vi "Multichannel Recording0.6.vi"() -> ()   [LabVIEW 2014]
uses:
  Multichannel Record/Enum State Typedef.ctl
  <vilib>/_DAQmxBase/Internals/DAQmxBase Create Channel (AI-Voltage-Basic).vi
  <vilib>/_DAQmxBase/Internals/DAQmxBase Timing (Sample Clock).vi
  <vilib>/_DAQmxBase/Internals/DAQmxBase Read (Analog 2D DBL NChan NSamp).vi
  Consumer Data_ Consumer Event Com.ctl
  Multichannel Record/Data Producer States.ctl
panel:
  in  "Display Size":T1(ring)
  out "Total Iterations Needed":dbl
  out "Read Data":i32
  out "Data Producer State":T2=enum."Default"
  out "Data Consumer State":T3=enum."Default"
  in  "Open Button":bool
  in  "Tab Control":T4(tab)
  in  "Amplifier Channel 0":T5 {"Amplifier Model" items=["Select a Model", "AM 1700", "BMA 200"]}
  out "Channel 0 Chart":waveform(dbl)(graph)
  in  "User Data Channel 0":T6
  in  "Use Channel 0":bool caption="In Use?"
  out "Channel 1 Chart":waveform(dbl)(graph)
  in  "User Data Channel 1":T6
  in  "Amplifier Channel 1":T5 {"Amplifier Model" items=["Select a Model", "AM 1700", "BMA 200"]}
  in  "Use Channel 1":bool caption="In Use?"
  out "Channel 2 Chart":waveform(dbl)(graph)
  in  "User Data Channel 2":T6
  in  "Amplifier Channel 2":T5 {"Amplifier Model" items=["Select a Model", "AM 1700", "BMA 200"]}
  in  "Use Channel 2":bool caption="In Use?"
  out "Channel 3 Chart":waveform(dbl)(graph)
  in  "User Data Channel 3":T6
  in  "Amplifier Channel 3":T5 {"Amplifier Model" items=["Select a Model", "AM 1700", "BMA 200"]}
  in  "Use Channel 3":bool caption="In Use?"
  out "Overview Chart":waveform(dbl)[](graph)
  in  "Stop Preview":bool
  in  "OK Button":bool
  out "Event State":T7
  in  "Clear Display":bool
  in  "Preview Button":bool
  out "Iterations Recorded":i32
  in  "Recording Time (seconds)":dbl
  in  "Sample Rate":i32=1000
  in  "Stop Button":bool
  out "Start Time hr/min":string
  out "Date mm/dd/yy":string
  in  "Exit Button":bool
  in  "Record Button":bool
  # "MSU EFISH Lab Multi-Channel Electronic Pulse Recorder"
  # "Must enter numbers into here before you start"
  # "Blue for On\nOrange for Off"
  # "DC"
  # "AC"
  # "Blue for AC and Orange for DC"
  # "Blue for On\nOrange for Off"
  # "DC"
  # "AC"
  # "Blue for AC and Orange for DC"
  # "Blue for On\nOrange for Off"
  # "DC"
  # "AC"
  # "Blue for AC and Orange for DC"
  # "Blue for On\nOrange for Off"
  # "DC"
  # "AC"
  # "Blue for AC and Orange for DC"
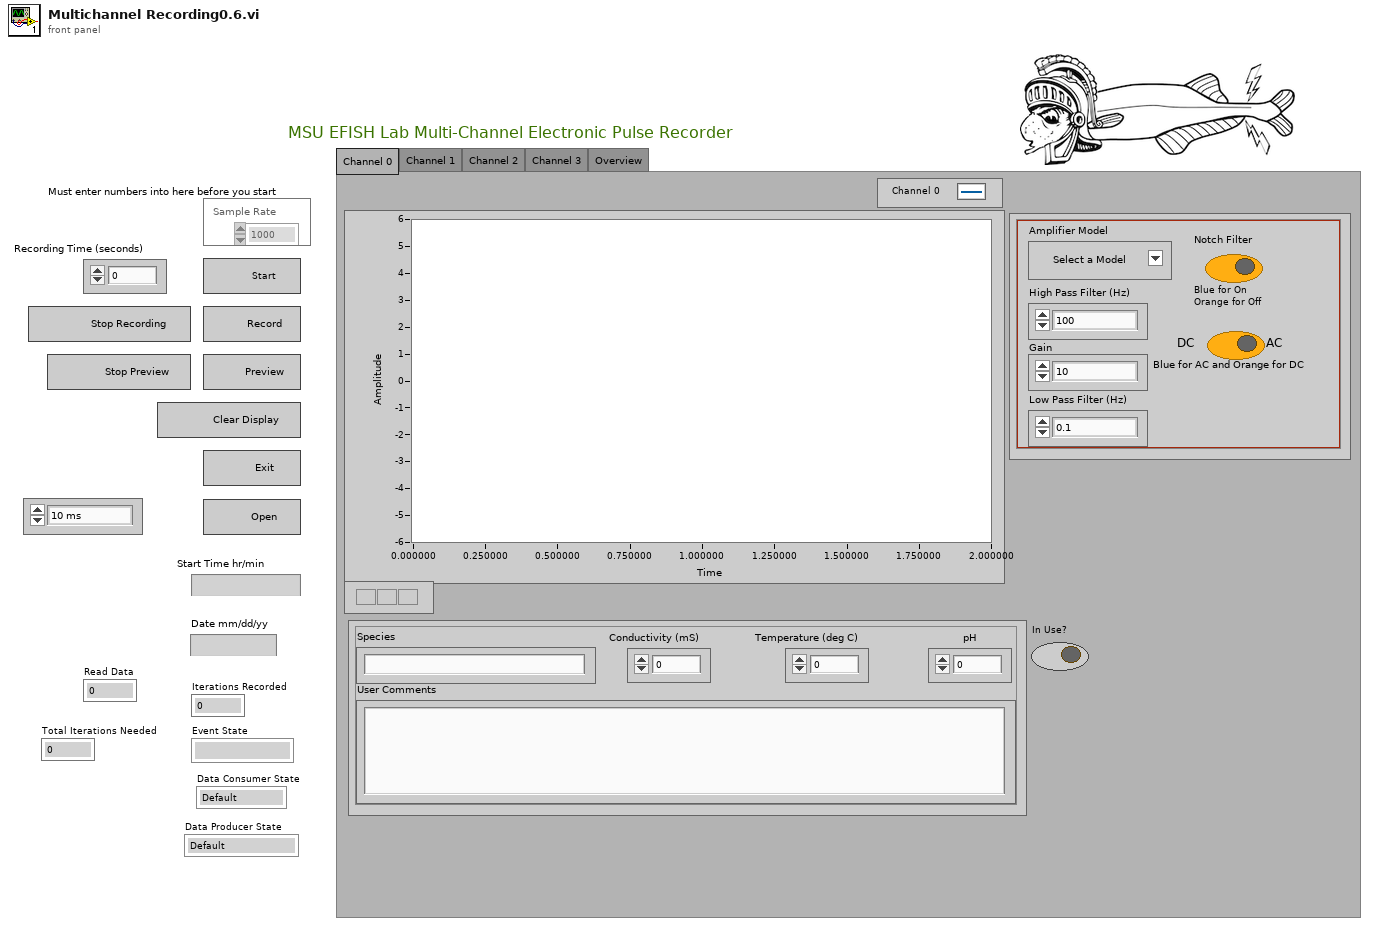
[diagram p1: front panel]
types:
  T1 = enum16{"10 ms", "100 ms", "1 Second", "10 sec", "30 sec"}
  T2 = typedef "Data Producer States.ctl" = enum16{"Read Data", "Set Sample Clock", "Default", "Exit", "Preview"}
  T3 = typedef "Consumer Data_ Consumer Event Com.ctl" = enum16{"Recording", "Create File", "Clear Memory", "Default", "End File", "Exit", "Set Sample Clock", "Preview"}
  T4 = enum32{"Channel 0", "Channel 1", "Channel 2", "Channel 3", "Overview"}
  T5 = cluster{"Low Pass Filter (Hz)":enum16{"0.1", "1", "3", "10", "30", "100", "300"}, "Gain ":enum16{"10", "20", "50", "100", "200", "500", "1000", "2k", "5k", "10k", "20k", "50k"}, "High Pass Filter (Hz)":enum16{"100", "500", "1000", "3000", "5000", "10,000", "20,000", "30,000", "50,000"}, "Notch Filter":bool, "Amplifier Model":u16, "AC/DC Switch":bool}
  T6 = cluster{"pH":dbl, "Conductivity (mS)":dbl, "Temperature (deg C)":dbl, "User Comments":string, "Species":string}
  T7 = typedef "Enum State Typedef.ctl" = enum16{"", "Open FIle", "Beginning State", "Set the Sample Clock", "Prepreview Handling", "Clear Display", "Preview Data", "Stop", "Exit", "Record", "Create File"}
  T8 = enum8{"Enabled", "Disabled", "Disabled and Grayed Out"}
  T9 = enum16{"Recording", "Create File", "Clear Memory", "Default"}
  T10 = cluster{"Refnum out":refnum<k34>, "Refnum out":refnum<k34>, "Refnum out":refnum<k34>, "Refnum out":refnum<k34>}
  T11 = cluster{"Use Channel 0":bool, "Use Channel 1":bool, "Use Channel 2":bool, "Use Channel 3":bool}
  T12 = cluster{"tdms file out":refnum<k34>, "tdms file out":refnum<k34>, "tdms file out":refnum<k34>, "tdms file out":refnum<k34>}
  T13 = cluster{"Waveform":waveform(dbl), "Waveform":waveform(dbl), "Waveform":waveform(dbl), "Waveform":waveform(dbl), waveform(dbl)[]}
  T14 = enum16{"Read Data", "Set Sample Clock", "Default", "Exit"}
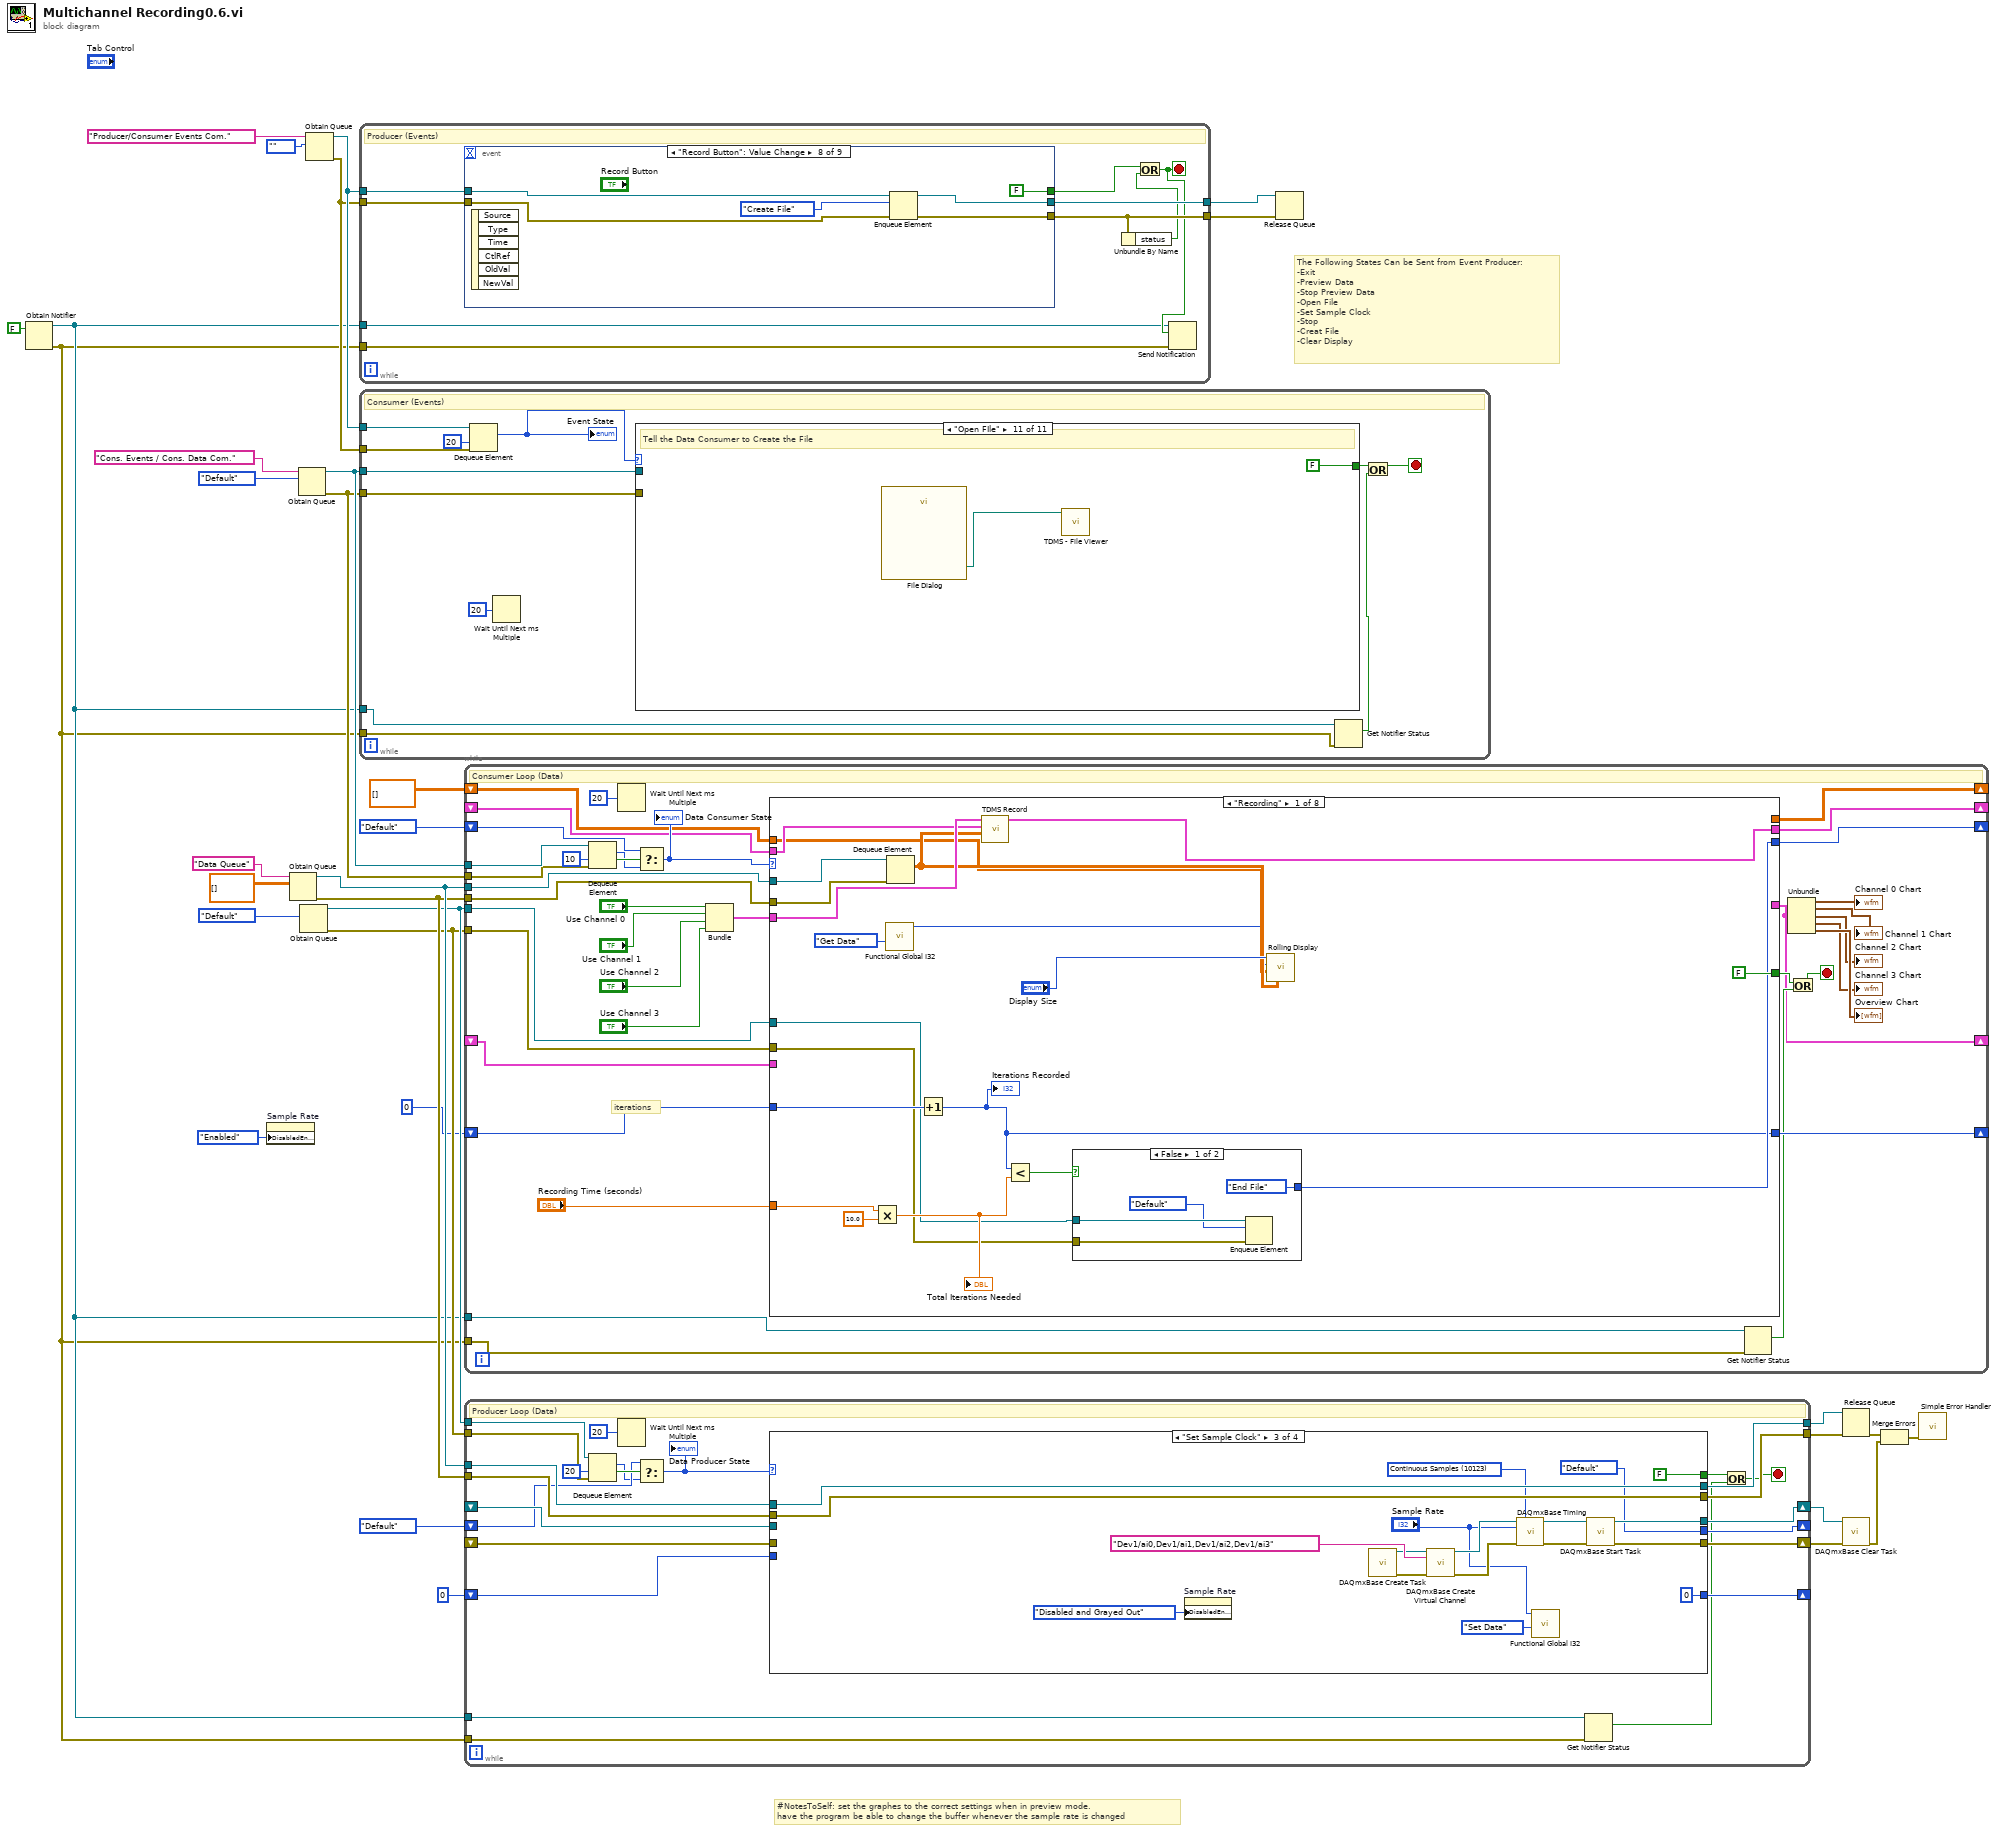
[diagram p0: block diagram]
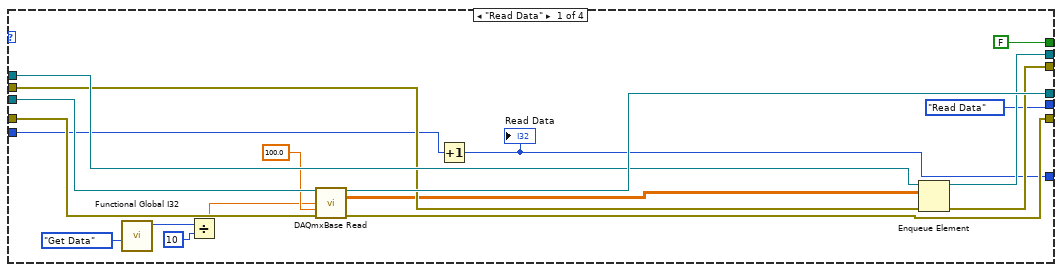
[diagram p2: hidden frame]
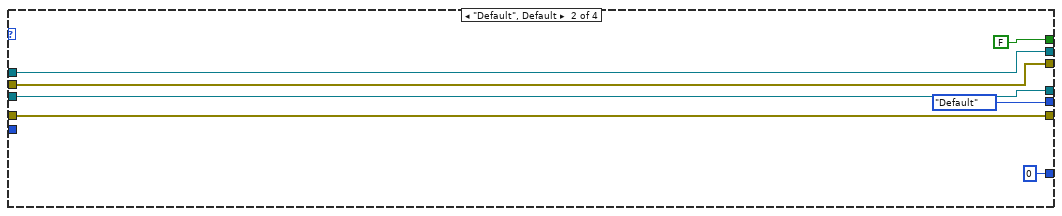
[diagram p3: hidden frame]
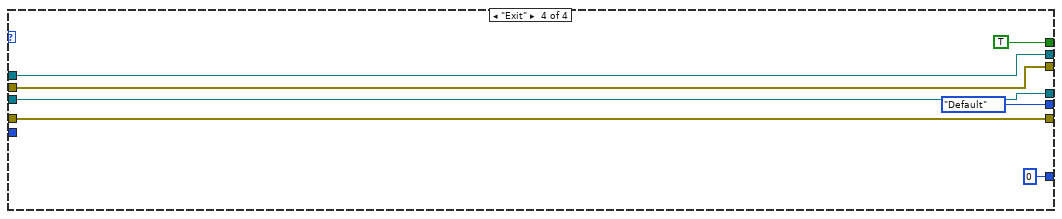
[diagram p4: hidden frame]
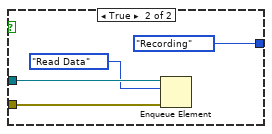
[diagram p5: hidden frame]
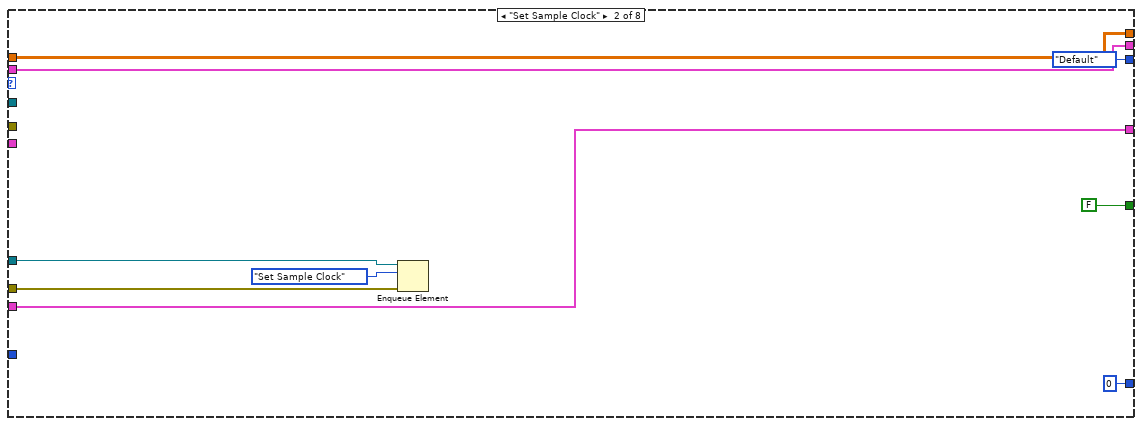
[diagram p6: hidden frame]
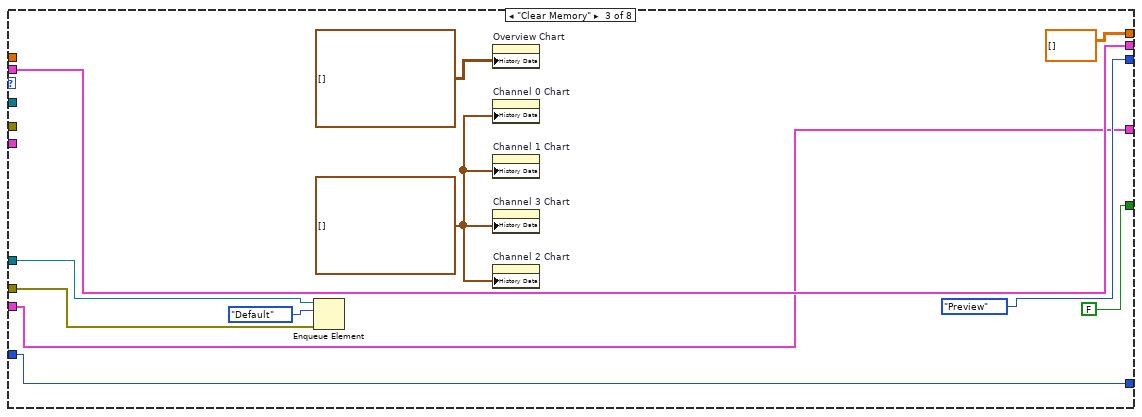
[diagram p7: hidden frame]
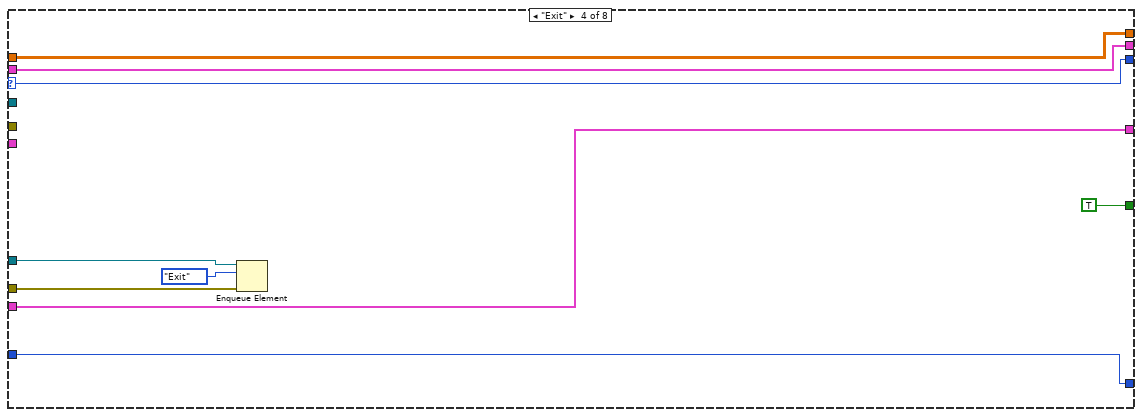
[diagram p8: hidden frame]
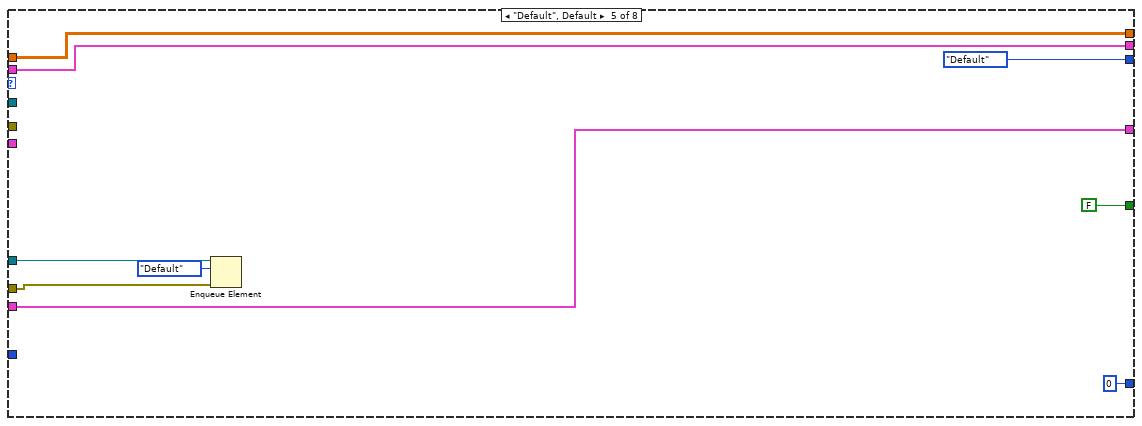
[diagram p9: hidden frame]
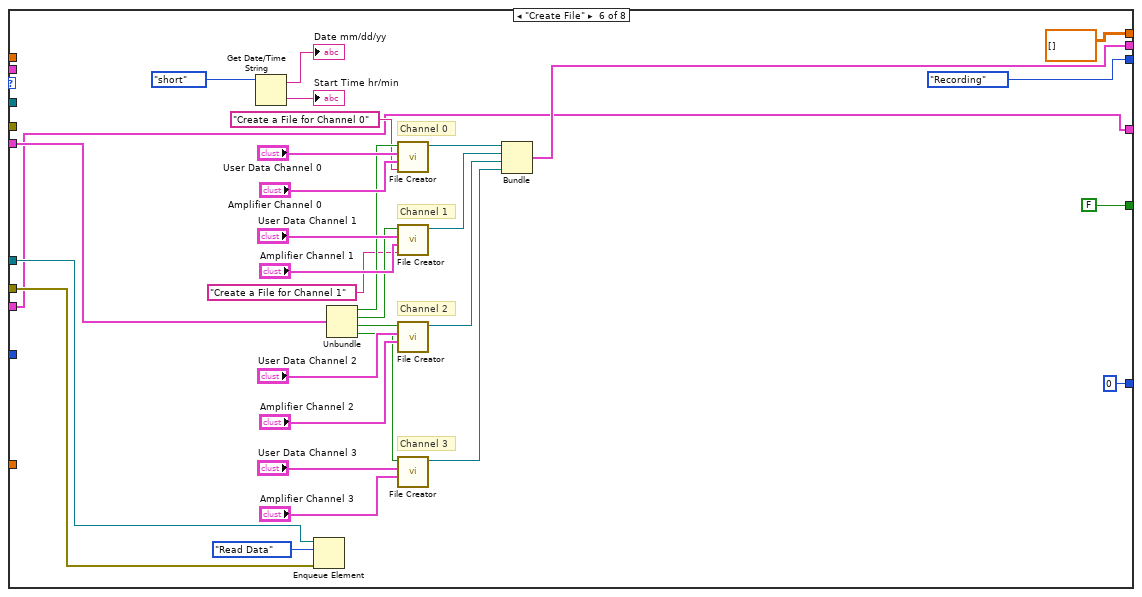
[diagram p10: hidden frame]
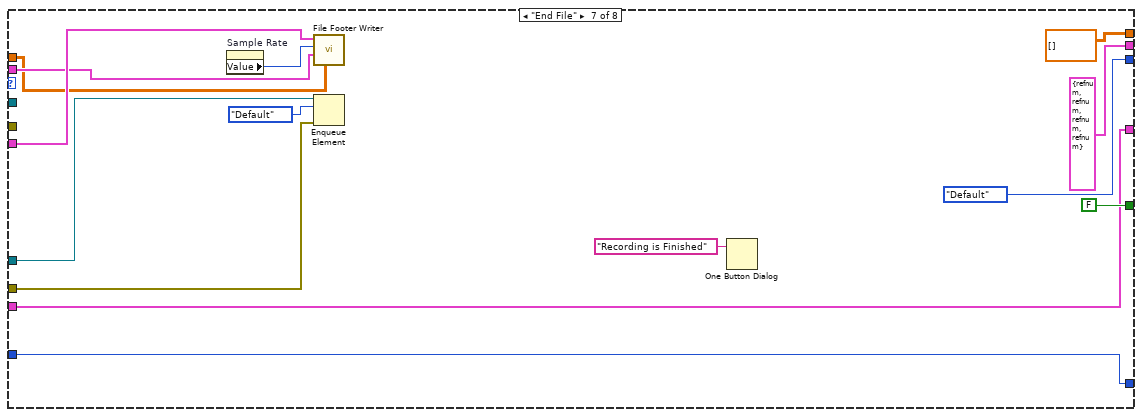
[diagram p11: hidden frame]
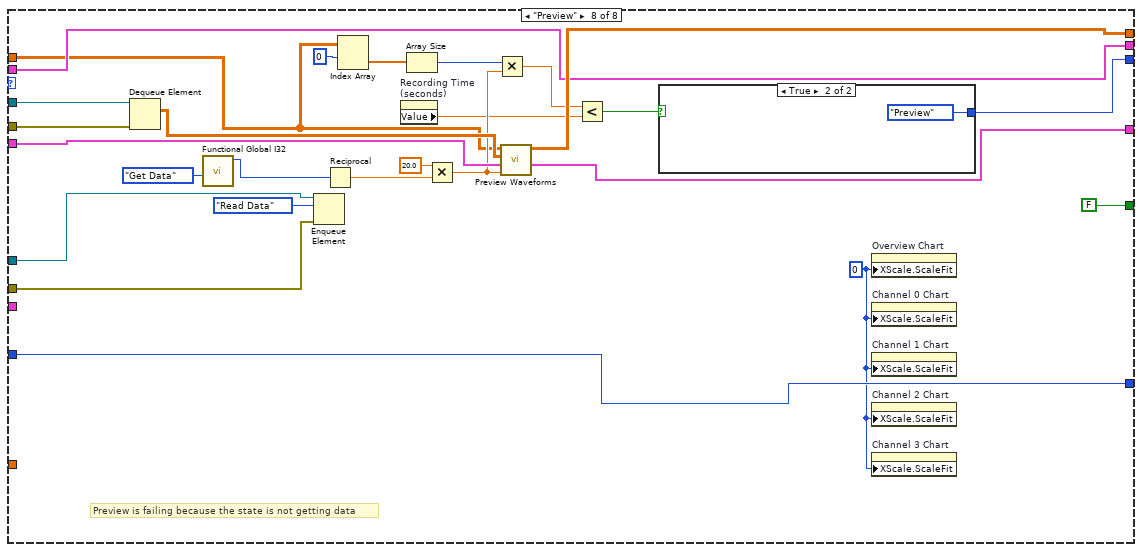
[diagram p12: hidden frame]
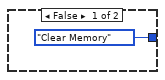
[diagram p13: hidden frame]
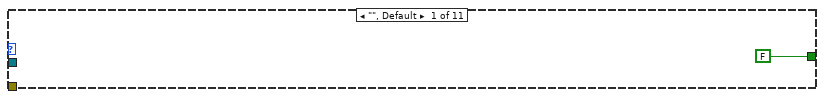
[diagram p14: hidden frame]
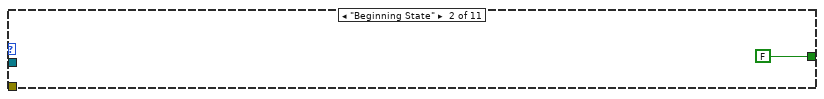
[diagram p15: hidden frame]
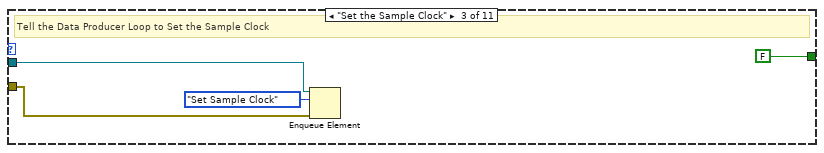
[diagram p16: hidden frame]
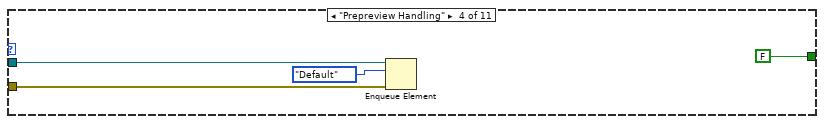
[diagram p17: hidden frame]
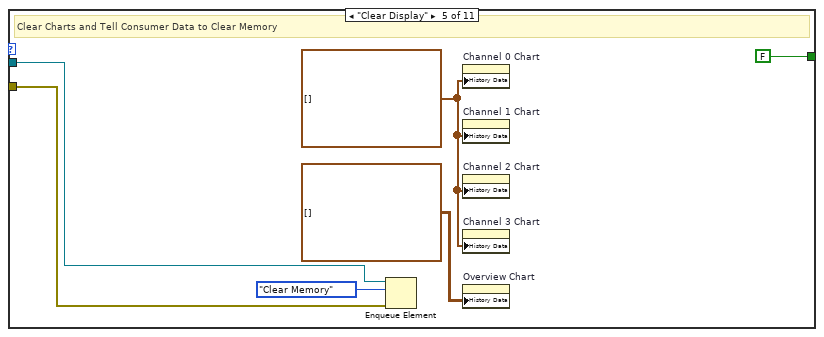
[diagram p18: hidden frame]
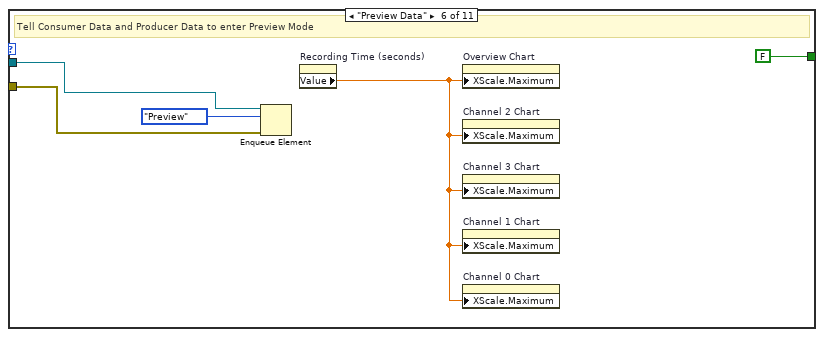
[diagram p19: hidden frame]
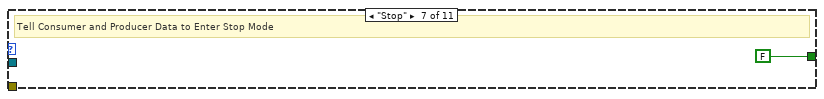
[diagram p20: hidden frame]
diagram:
  # "#NotesToSelf: set the graphes to the correct settings when in preview mode.\nhave the program be able to change the buffer whenever the sample rate is changed"
  # "The Following States Can be Sent from Event Producer:\n-Exit\n-Preview Data\n-Stop Preview Data\n-Open File\n-Set Sample Clock\n-Stop\n-Creat File\n-Clear Display"
  n1 = Obtain Notifier(notification data type=FALSE) -> (notifier out=w2:refnum<notifier>, error out=w1:errorcluster)  [unwired: 3 in, 1 out]
  n2 = property on="Sample Rate" class="DigNum (strict)"("DisabledEnum"=T8."Enabled" ("Disabled")) -> ()  [unwired: 2 in, 2 out]
  n3 = Obtain Queue(name (unnamed)="Data Queue", element data type=dbl[][] []) -> (queue out=w28:refnum<queue>, error out=w27:errorcluster)  [unwired: 3 in, 1 out]
  n4 = Obtain Queue(name (unnamed)="Cons. Events / Cons. Data Com.", element data type=Consumer_Data__Consumer_Event_Com."Default") -> (queue out=w20:refnum<queue>, error out=w19:errorcluster)  [unwired: 3 in, 1 out]
  n5 = Obtain Queue(element data type=Data_Producer_States."Default") -> (queue out=w9:refnum<queue>, error out=w8:errorcluster)  [unwired: 4 in, 1 out]
  n6 = Obtain Queue(name (unnamed)="Producer/Consumer Events Com.", element data type=Enum_State_Typedef."" ("State")) -> (queue out=w32:refnum<queue>, error out=w31:errorcluster)  [unwired: 3 in, 1 out]
  n7 = while {
    tunnel: w32 -> [w42]
    tunnel: w31 -> [w41]
    tunnel: [w40] -> w26
    tunnel: [w39] -> w25
    tunnel: w2 -> [w35]
    tunnel: w1 -> [w34]
    stop <- w36 stop-if-true
    # "Producer (Events)"
    n8 = event shown="[7] \"Record Button\": Value Change" {
      selector: _ -> [_ _ _ _ _ _ _ _ _]
      dyn-events: _ -> [_ _ _ _ _ _ _ _ _]
      timeout: _ -> [_ _ _ _ _ _ _ _ _]
      tunnel: [FALSE ("Exit Button") "Exit Button" FALSE ("Exit Button") FALSE ("Exit Button") FALSE ("Exit Button") FALSE ("Exit Button") FALSE ("Exit Button") FALSE ("Exit Button") FALSE ("Exit Button")] -> w38
      tunnel: w42 -> [w44 w50 w57 w63 w69 w75 w81 w87 w93]
      tunnel: w41 -> [w43 w49 w56 w62 w68 w74 w80 w86 w92]
      tunnel: [w44 w47 w53 w59 w65 w71 w77 w83 w89] -> w40
      tunnel: [w43 w46 w52 w58 w64 w70 w76 w82 w88] -> w39
      event Timeout {
        n9 = event-data() -> ()  [unwired: 1 in, 3 out]
      }
      event "Exit Button": Value Change {
        n10 = event-data() -> ()  [unwired: 1 in, 1 out]
        n11 = Enqueue Element(queue=w50, element=Enum_State_Typedef."Exit", error in (no error)=w49) -> (queue out=w47:refnum<queue>, error out=w46:errorcluster)  [unwired: 1 in, 1 out]
      }
      event "Preview Button": Value Change {
        n12 = event-data() -> ()  [unwired: 1 in, 6 out]
        n13 = Enqueue Element(queue=w57, element=Enum_State_Typedef."Preview Data", error in (no error)=w56) -> (queue out=w53:refnum<queue>, error out=w52:errorcluster)  [unwired: 1 in, 1 out]
      }
      event "Stop Preview": Value Change {
        n14 = event-data() -> ()  [unwired: 1 in, 6 out]
        n15 = Enqueue Element(queue=w63, element=Enum_State_Typedef."Prepreview Handling", error in (no error)=w62) -> (queue out=w59:refnum<queue>, error out=w58:errorcluster)  [unwired: 1 in, 1 out]
      }
      event "Open Button": Value Change {
        n16 = event-data() -> ()  [unwired: 1 in, 6 out]
        n17 = Enqueue Element(queue=w69, element=Enum_State_Typedef."Open FIle", error in (no error)=w68) -> (queue out=w65:refnum<queue>, error out=w64:errorcluster)  [unwired: 1 in, 1 out]
      }
      event "OK Button": Value Change {
        n18 = event-data() -> ()  [unwired: 1 in, 6 out]
        n19 = Enqueue Element(queue=w75, element=Enum_State_Typedef."Set the Sample Clock", error in (no error)=w74) -> (queue out=w71:refnum<queue>, error out=w70:errorcluster)  [unwired: 1 in, 1 out]
      }
      event "Stop Button": Value Change {
        n20 = event-data() -> ()  [unwired: 1 in, 6 out]
        n21 = Enqueue Element(queue=w81, element=Enum_State_Typedef."Stop", error in (no error)=w80) -> (queue out=w77:refnum<queue>, error out=w76:errorcluster)  [unwired: 1 in, 1 out]
      }
      event "Record Button": Value Change {
        n22 = event-data() -> ()  [unwired: 1 in, 6 out]
        n23 = Enqueue Element(queue=w87, element=Enum_State_Typedef."Create File", error in (no error)=w86) -> (queue out=w83:refnum<queue>, error out=w82:errorcluster)  [unwired: 1 in, 1 out]
      }
      event "Clear Display": Value Change {
        n24 = event-data() -> ()  [unwired: 1 in, 6 out]
        n25 = Enqueue Element(queue=w93, element=Enum_State_Typedef."Clear Display", error in (no error)=w92) -> (queue out=w89:refnum<queue>, error out=w88:errorcluster)  [unwired: 1 in, 1 out]
      }
    }
    n26 = Unbundle By Name(w39) -> ("status"=w37:bool)
    n27 = Or(x=w38, y=w37) -> (x .or. y?=w36:bool)
    n28 = Send Notification(notification=w36, notifier=w35, error in (no error)=w34) -> ()  [unwired: 2 out]
  }
  n29 = while {
    tunnel: w32 -> [w105]
    tunnel: w31 -> [w104]
    tunnel: w20 -> [w103]
    tunnel: w19 -> [w102]
    tunnel: w2 -> [w97]
    tunnel: w1 -> [w96]
    stop <- w95 stop-if-true
    # "Consumer (Events)"
    n30 = Dequeue Element(queue=w105, timeout in ms (-1)=20, error in (no error)=w104) -> (element=w100:T7)  [unwired: 3 out]
    "Event State" <- w100
    n31 = Wait Until Next ms Multiple(millisecond multiple=u32 20) -> ()  [unwired: 1 out]
    n32 = case shown="\"Open FIle\"" w100 {
      tunnel: w103 -> [_ _ w110 w114 w118 w124 _ w131 _ w136 _]
      tunnel: w102 -> [_ _ w109 w113 w117 w123 _ w130 _ w135 _]
      tunnel: [FALSE FALSE FALSE FALSE FALSE FALSE FALSE TRUE FALSE FALSE FALSE] -> w101
      frame "", Default {
      }
      frame "Beginning State" {
      }
      frame "Set the Sample Clock" {
        # "Tell the Data Producer Loop to Set the Sample Clock"
        n33 = Enqueue Element(queue=w110, element=Consumer_Data__Consumer_Event_Com."Set Sample Clock", error in (no error)=w109) -> ()  [unwired: 1 in, 3 out]
      }
      frame "Prepreview Handling" {
        n34 = Enqueue Element(queue=w114, element=Consumer_Data__Consumer_Event_Com."Default", error in (no error)=w113) -> ()  [unwired: 1 in, 3 out]
      }
      frame "Clear Display" {
        w120 = waveform(dbl)[] [] ("History Data")
        # "Clear Charts and Tell Consumer Data to Clear Memory"
        n35 = Enqueue Element(queue=w118, element=Consumer_Data__Consumer_Event_Com."Clear Memory", error in (no error)=w117) -> ()  [unwired: 1 in, 3 out]
        n36 = property on="Channel 0 Chart" class="WFChart (strict)"("History Data"=w120) -> ()  [unwired: 2 in, 2 out]
        n37 = property on="Channel 1 Chart" class="WFChart (strict)"("History Data"=w120) -> ()  [unwired: 2 in, 2 out]
        n38 = property on="Channel 2 Chart" class="WFChart (strict)"("History Data"=w120) -> ()  [unwired: 2 in, 2 out]
        n39 = property on="Channel 3 Chart" class="WFChart (strict)"("History Data"=w120) -> ()  [unwired: 2 in, 2 out]
        n40 = property on="Overview Chart" class="WFChart (strict)"("History Data"=waveform(dbl)[][] []) -> ()  [unwired: 2 in, 2 out]
      }
      frame "Preview Data" {
        # "Tell Consumer Data and Producer Data to enter Preview Mode"
        n41 = Enqueue Element(queue=w124, element=Consumer_Data__Consumer_Event_Com."Preview", error in (no error)=w123) -> ()  [unwired: 1 in, 3 out]
        n42 = property on="Recording Time (seconds)" class="DigNum (strict)"() -> ("Value"=w125:dbl)  [unwired: 2 in, 2 out]
        n43 = property on="Overview Chart" class="WFChart (strict)"("XScale.Maximum"=w125) -> ()  [unwired: 2 in, 2 out]
        n44 = property on="Channel 2 Chart" class="WFChart (strict)"("XScale.Maximum"=w125) -> ()  [unwired: 2 in, 2 out]
        n45 = property on="Channel 3 Chart" class="WFChart (strict)"("XScale.Maximum"=w125) -> ()  [unwired: 2 in, 2 out]
        n46 = property on="Channel 1 Chart" class="WFChart (strict)"("XScale.Maximum"=w125) -> ()  [unwired: 2 in, 2 out]
        n47 = property on="Channel 0 Chart" class="WFChart (strict)"("XScale.Maximum"=w125) -> ()  [unwired: 2 in, 2 out]
      }
      frame "Stop" {
        # "Tell Consumer and Producer Data to Enter Stop Mode"
      }
      frame "Exit" {
        # "Tell Producer and Consumer Data to end themselves then End the Program"
        n48 = Enqueue Element(queue=w131, element=Consumer_Data__Consumer_Event_Com."Exit", error in (no error)=w130) -> ()  [unwired: 1 in, 3 out]
      }
      frame "Record" {
        # "(I dont think that this case will exist)"
      }
      frame "Create File" {
        w133 = u8 2 ("X Scale.Scale Fit")
        # "Let Consumer Data Create File"
        n49 = Enqueue Element(queue=w136, element=Consumer_Data__Consumer_Event_Com."Create File", error in (no error)=w135) -> ()  [unwired: 1 in, 3 out]
        n50 = property on="Overview Chart" class="WFChart (strict)"("XScale.ScaleFit"=w133) -> ()  [unwired: 2 in, 2 out]
        n51 = property on="Channel 3 Chart" class="WFChart (strict)"("XScale.ScaleFit"=w133) -> ()  [unwired: 2 in, 2 out]
        n52 = property on="Channel 2 Chart" class="WFChart (strict)"("XScale.ScaleFit"=w133) -> ()  [unwired: 2 in, 2 out]
        n53 = property on="Channel 1 Chart" class="WFChart (strict)"("XScale.ScaleFit"=w133) -> ()  [unwired: 2 in, 2 out]
        n54 = property on="Channel 0 Chart" class="WFChart (strict)"("XScale.ScaleFit"=w133) -> ()  [unwired: 2 in, 2 out]
      }
      frame "Open FIle" {
        # "Tell the Data Consumer to Create the File"
        n55 = call "File Dialog"() -> ("selected path"=w138:path)  [unwired: 12 in, 3 out]
        n56 = call <vilib>:"TDMS - File Viewer.vi"("file path"=w138) -> ()  [unwired: 5 in, 2 out]
      }
    }
    n57 = Get Notifier Status(notifier=w97, error in (no error)=w96) -> (current notification=w94:bool)  [unwired: 4 out]
    n58 = Or(x=w101, y=w94) -> (x .or. y?=w95:bool)
  }
  n59 = while {
    tunnel: w28 -> [w169]
    tunnel: w27 -> [w168]
    tunnel: w20 -> [w176]
    tunnel: w19 -> [w175]
    shift-right: [w170] -> _
    shift-left: Consumer_Data__Consumer_Event_Com."Default" -> [w171]
    shift-right: [w164] -> _
    shift-left: dbl[][] [] -> [w167]
    shift-right: [w163] -> _
    shift-left: _ -> [w162]
    tunnel: w9 -> [w160]
    tunnel: w8 -> [w159]
    shift-right: [w155] -> _
    shift-left: 0 -> [w157]
    tunnel: w2 -> [w149]
    tunnel: w1 -> [w148]
    shift-right: [w141] -> _
    shift-left: _ -> [w140]
    stop <- w151 stop-if-true
    # "iterations"
    # "Consumer Loop (Data)"
    n60 = Dequeue Element(queue=w176, timeout in ms (-1)=10, error in (no error)=w175) -> (element=w173:T3, timed out?=w174:bool)  [unwired: 2 out]
    n61 = Wait Until Next ms Multiple(millisecond multiple=u32 20) -> ()  [unwired: 1 out]
    n62 = Select(t=w171, s=w174, f=w173) -> (s? t:f=w172:T3)
    "Data Consumer State" <- w172
    n63 = Bundle("Use Channel 0"="Use Channel 0", "Use Channel 1"="Use Channel 1", "Use Channel 2"="Use Channel 2", "Use Channel 3"="Use Channel 3") -> (w165:T11)  [unwired: 1 in]
    n64 = case shown="\"Recording\"" w172 {
      selector: w172 -> [_ _ _ w231 _ _ _ _]
      tunnel: [w186 Consumer_Data__Consumer_Event_Com."Default" Consumer_Data__Consumer_Event_Com."Preview" w231 T9."Default" Consumer_Data__Consumer_Event_Com."Recording" Consumer_Data__Consumer_Event_Com."Default" w297] -> w170
      tunnel: w169 -> [w195 _ _ _ _ _ _ w313]
      tunnel: w168 -> [w194 _ _ _ _ _ _ w312]
      tunnel: [FALSE FALSE FALSE TRUE FALSE FALSE FALSE FALSE] -> w150
      tunnel: w167 -> [w178 w210 _ w232 w240 _ w285 w304]
      tunnel: w165 -> [w193 _ _ _ _ w267 w287 w310]
      tunnel: [_ w210 dbl[][] [] ("Output Decimated Data") w232 w240 dbl[][] [] ("Output Decimated Data") dbl[][] [] ("Output Data") w307] -> w164
      tunnel: [w192 w209 w221 w230 w239 w250 T10 {"Refnum out"=refnum, "Refnum out"=refnum, "Refnum out"=refnum, "Refnum out"=refnum} ("Output TDMS File Cluster") w306] -> w163
      tunnel: w162 -> [w182 w209 w221 w230 w239 _ w286 w306]
      tunnel: w160 -> [w185 w213 w218 w229 w237 w249 w279 w295]
      tunnel: w159 -> [w184 w212 w217 w228 w236 w248 w278 w294]
      tunnel: w157 -> [w191 _ w215 w226 _ _ w276 w292]
      tunnel: "Recording Time (seconds)" -> [w190 _ _ _ _ _ _ _]
      tunnel: [w183 0 w215 w226 0 0 w276 w292] -> w155
      tunnel: [_ w205 w214 w225 w234 w243 w274 w288] -> w141
      tunnel: w140 -> [_ w205 w214 w225 w234 w243 w274 _]
      frame "Recording" {
        n65 = Multiply(x=w190, y=10.0) -> (x*y=w188:dbl)
        "Total Iterations Needed" <- w188
        n66 = call "Functional Global I32.vi"("Enum"=enum16{"Set Data", "Get Data"}."Get Data") -> ("Integer"=w177:i32)  [unwired: 10 in]
        n67 = Dequeue Element(queue=w195, error in (no error)=w194) -> (element=w179:dbl[][])  [unwired: 1 in, 3 out]
        n68 = Increment(x=w191) -> (x+1=w183:i32)
        "Iterations Recorded" <- w183
        n69 = call "TDMS Record.vi"("Data"=w179, "Input TDMS File Cluster"=w182, "In Use Cluster"=w193) -> ("Output TDMS File Cluster"=w192:T12)  [unwired: 8 in]
        n70 = Less?(x=w183, y=w188) -> (x < y?=w187:bool)
        n71 = case shown="False" w187 {
          tunnel: [Consumer_Data__Consumer_Event_Com."End File" Consumer_Data__Consumer_Event_Com."Recording"] -> w186
          tunnel: w185 -> [w199 w203]
          tunnel: w184 -> [w198 w202]
          frame False {
            n72 = Enqueue Element(queue=w199, element=Data_Producer_States."Default", error in (no error)=w198) -> ()  [unwired: 1 in, 3 out]
          }
          frame True {
            n73 = Enqueue Element(queue=w203, element=Data_Producer_States."Read Data", error in (no error)=w202) -> ()  [unwired: 1 in, 3 out]
          }
        }
        n74 = call "Rolling Display.vi"("Input Data"=w179, "Old Data"=w178, "Sample Rate"=w177, "Display Size"="Display Size") -> ()  [unwired: 8 in]
      }
      frame "Set Sample Clock" {
        n75 = Enqueue Element(queue=w213, element=Data_Producer_States."Set Sample Clock", error in (no error)=w212) -> ()  [unwired: 1 in, 3 out]
      }
      frame "Clear Memory" {
        w219 = waveform(dbl)[] [] ("History Data")
        n76 = Enqueue Element(queue=w218, element=Data_Producer_States."Default", error in (no error)=w217) -> ()  [unwired: 1 in, 3 out]
        n77 = property on="Overview Chart" class="WFChart (strict)"("History Data"=waveform(dbl)[][] []) -> ()  [unwired: 2 in, 2 out]
        n78 = property on="Channel 0 Chart" class="WFChart (strict)"("History Data"=w219) -> ()  [unwired: 2 in, 2 out]
        n79 = property on="Channel 1 Chart" class="WFChart (strict)"("History Data"=w219) -> ()  [unwired: 2 in, 2 out]
        n80 = property on="Channel 3 Chart" class="WFChart (strict)"("History Data"=w219) -> ()  [unwired: 2 in, 2 out]
        n81 = property on="Channel 2 Chart" class="WFChart (strict)"("History Data"=w219) -> ()  [unwired: 2 in, 2 out]
      }
      frame "Exit" {
        n82 = Enqueue Element(queue=w229, element=Data_Producer_States."Exit", error in (no error)=w228) -> ()  [unwired: 1 in, 3 out]
      }
      frame "Default", Default {
        n83 = Enqueue Element(queue=w237, element=Data_Producer_States."Default", error in (no error)=w236) -> ()  [unwired: 1 in, 3 out]
      }
      frame "Create File" {
        # "Channel 3"
        # "Channel 2"
        # "Channel 1"
        # "Channel 0"
        n84 = Get Date/Time String(date format (0)=enum16{"short", "long", "abbreviated"}."short") -> (date string=→"Date mm/dd/yy":string, time string=→"Start Time hr/min":string)  [unwired: 2 in]
        n85 = Enqueue Element(queue=w249, element=Data_Producer_States."Read Data", error in (no error)=w248) -> ()  [unwired: 1 in, 3 out]
        n86 = Unbundle(w267) -> ("Use Channel 0"=w260:bool, "Use Channel 1"=w259:bool, "Use Channel 2"=w258:bool, "Use Channel 3"=w257:bool)
        n87 = call "File Creator.vi"("prompt"="Create a File for Channel 0", "Amplifier Channel 1"="Amplifier Channel 0", "User Data Channel 1"="User Data Channel 0", "Use Channel in"=w260) -> ("Refnum out"=w256:refnum<k34>)  [unwired: 7 in]
        n88 = call "File Creator.vi"("prompt"="Create a File for Channel 1", "Amplifier Channel 1"="Amplifier Channel 1", "User Data Channel 1"="User Data Channel 1", "Use Channel in"=w259) -> ("Refnum out"=w255:refnum<k34>)  [unwired: 7 in]
        n89 = call "File Creator.vi"("Amplifier Channel 1"="Amplifier Channel 2", "User Data Channel 1"="User Data Channel 2", "Use Channel in"=w258) -> ("Refnum out"=w254:refnum<k34>)  [unwired: 8 in]
        n90 = call "File Creator.vi"("Amplifier Channel 1"="Amplifier Channel 3", "User Data Channel 1"="User Data Channel 3", "Use Channel in"=w257) -> ("Refnum out"=w253:refnum<k34>)  [unwired: 8 in]
        n91 = Bundle("Refnum out"=w256, "Refnum out"=w255, "Refnum out"=w254, "Refnum out"=w253) -> (w250:T10)  [unwired: 1 in]
      }
      frame "End File" {
        n92 = property on="Sample Rate" class="DigNum (strict)"() -> ("Value"=w284:i32)  [unwired: 2 in, 2 out]
        n93 = call "File Footer Writer.vi"("Old Data"=w285, "TDMS File Cluster"=w286, "Sample Rate"=w284, "In Use Cluster"=w287) -> ()  [unwired: 8 in]
        n94 = Enqueue Element(queue=w279, element=Data_Producer_States."Default", error in (no error)=w278) -> ()  [unwired: 1 in, 3 out]
        n95 = One Button Dialog(message="Recording is Finished") -> ()  [unwired: 1 in, 1 out]
      }
      frame "Preview" {
        w289 = u8 0 ("X Scale.Scale Fit")
        # "Preview is failing because the state is not getting data"
        n96 = Dequeue Element(queue=w313, error in (no error)=w312) -> (element=w311:dbl[][])  [unwired: 1 in, 3 out]
        n97 = call "Functional Global I32.vi"("Enum"=enum16{"Set Data", "Get Data"}."Get Data") -> ("Integer"=w290:i32)  [unwired: 10 in]
        n98 = Enqueue Element(queue=w295, element=Data_Producer_States."Read Data", error in (no error)=w294) -> ()  [unwired: 1 in, 3 out]
        n99 = Reciprocal(x=w290) -> (1/x=w309:dbl)
        n100 = Index Array(array=w304, index (row)=0) -> (element=w302:dbl[])  [unwired: 1 in]
        n101 = property on="Recording Time (seconds)" class="DigNum (strict)"() -> ("Value"=w299:dbl)  [unwired: 2 in, 2 out]
        n102 = Array Size(array=w302) -> (size(s)=w301:i32)
        n103 = Multiply(x=20.0, y=w309) -> (x*y=w305:dbl)
        n104 = Multiply(x=w301, y=w305) -> (x*y=w300:dbl)
        n105 = call "Preview Waveforms.vi"("Change in Time"=w305, "In Use Cluster"=w310, "Input Read Data"=w311, "Input Decimated Data"=w304) -> ("Output Waveform Cluster"=w288:T13, "Output Data"=w307:dbl[][])  [unwired: 6 in]
        n106 = Less?(x=w300, y=w299) -> (x < y?=w298:bool)
        n107 = case shown="True" w298 {
          tunnel: [Consumer_Data__Consumer_Event_Com."Clear Memory" Consumer_Data__Consumer_Event_Com."Preview"] -> w297
          frame False {
          }
          frame True {
          }
        }
        n108 = property on="Overview Chart" class="WFChart (strict)"("XScale.ScaleFit"=w289) -> ()  [unwired: 2 in, 2 out]
        n109 = property on="Channel 0 Chart" class="WFChart (strict)"("XScale.ScaleFit"=w289) -> ()  [unwired: 2 in, 2 out]
        n110 = property on="Channel 1 Chart" class="WFChart (strict)"("XScale.ScaleFit"=w289) -> ()  [unwired: 2 in, 2 out]
        n111 = property on="Channel 2 Chart" class="WFChart (strict)"("XScale.ScaleFit"=w289) -> ()  [unwired: 2 in, 2 out]
        n112 = property on="Channel 3 Chart" class="WFChart (strict)"("XScale.ScaleFit"=w289) -> ()  [unwired: 2 in, 2 out]
      }
    }
    n113 = Get Notifier Status(notifier=w149, error in (no error)=w148) -> (current notification=w147:bool)  [unwired: 4 out]
    n114 = Unbundle(w141) -> ("Waveform"=→"Channel 0 Chart":waveform(dbl), "Waveform"=→"Channel 1 Chart":waveform(dbl), "Waveform"=→"Channel 2 Chart":waveform(dbl), "Waveform"=→"Channel 3 Chart":waveform(dbl), →"Overview Chart":waveform(dbl)[])
    n115 = Or(x=w150, y=w147) -> (x .or. y?=w151:bool)
  }
  n116 = while {
    tunnel: w28 -> [w339]
    tunnel: w27 -> [w336]
    tunnel: [w338] -> w24
    tunnel: [w337] -> w23
    shift-right: [w324] -> _
    shift-left: Data_Producer_States."Default" -> [w317]
    shift-right: [w335] -> w17
    shift-left: _ -> [w333]
    shift-right: [w334] -> w16
    shift-left: _ -> [w332]
    tunnel: w9 -> [w329]
    tunnel: w8 -> [w328]
    shift-right: [w322] -> _
    shift-left: 0 -> [w323]
    tunnel: w2 -> [w319]
    tunnel: w1 -> [w318]
    stop <- w321 stop-if-true
    # "Producer Loop (Data)"
    n117 = Dequeue Element(queue=w329, timeout in ms (-1)=20, error in (no error)=w328) -> (element=w316:T2, timed out?=w327:bool)  [unwired: 2 out]
    n118 = Wait Until Next ms Multiple(millisecond multiple=u32 20) -> ()  [unwired: 1 out]
    n119 = Select(t=w317, s=w327, f=w316) -> (s? t:f=w326:T2)
    "Data Producer State" <- w326
    n120 = case shown="\"Set Sample Clock\"" w326 {
      tunnel: w339 -> [w353 w364 w373 w385]
      tunnel: [w351 w364 w373 w385] -> w338
      tunnel: [w350 w363 w372 w386] -> w337
      tunnel: w336 -> [w352 w363 w372 w386]
      tunnel: [w355 w362 w375 w387] -> w335
      tunnel: [w354 w361 w374 w388] -> w334
      tunnel: w333 -> [w357 w362 _ w387]
      tunnel: w332 -> [w356 w361 _ w388]
      tunnel: [FALSE FALSE FALSE TRUE] -> w330
      tunnel: [Data_Producer_States."Read Data" Data_Producer_States."Default" T14."Default" Data_Producer_States."Default"] -> w324
      tunnel: w323 -> [w346 _ _ _]
      tunnel: [w345 0 0 0] -> w322
      frame "Read Data" {
        n121 = call "Functional Global I32.vi"("Enum"=enum16{"Set Data", "Get Data"}."Get Data") -> ("Integer"=w342:i32)  [unwired: 10 in]
        n122 = Divide(x=w342, y=10) -> (x/y=w341:dbl)
        n123 = call-poly <vilib>:"DAQmxBase Read.vi"("task/channels in"=w357, "number of samples per channel"=w341, "timeout"=100.0, "error in"=w356) -> ("task out"=w355:refnum<k21>, "data"=w340:dbl[][], "error out"=w354:errorcluster)  [unwired: 9 in]
        n124 = Increment(x=w346) -> (x+1=w345:i32)
        "Read Data" <- w345
        n125 = Enqueue Element(queue=w353, element=w340, error in (no error)=w352) -> (queue out=w351:refnum<queue>, error out=w350:errorcluster)  [unwired: 1 in, 1 out]
      }
      frame "Default", Default {
      }
      frame "Set Sample Clock" {
        w365 = 10123 items=["Finite Samples"=10178, "Continuous Samples"=10123, "Hardware Timed Single Point"=12522] ("sample mode")
        n126 = property on="Sample Rate" class="DigNum (strict)"("DisabledEnum"=T8."Disabled and Grayed Out" ("Disabled")) -> ()  [unwired: 2 in, 2 out]
        n127 = call <vilib>:"DAQmxBase Create Task.vi"() -> ("task out"=w381:refnum<k21>, "error out"=w380:errorcluster)  [unwired: 14 in]
        n128 = call-poly <vilib>:"DAQmxBase Create Virtual Channel.vi"("task in"=w381, "physical channels"=tag "Dev1/ai0,Dev1/ai1,Dev1/ai2,Dev1/ai3", "error in"=w380) -> ("task out"=w378:refnum<k21>, "error out"=w379:errorcluster)  [unwired: 11 in]
        n129 = call-poly <vilib>:"DAQmxBase Timing.vi"("task/channels in"=w378, "sample mode"=w365, "rate"="Sample Rate", "error in"=w379) -> ("task out"=w377:refnum<k21>, "error out"=w376:errorcluster)  [unwired: 10 in]
        n130 = call "Functional Global I32.vi"("Enum"=enum16{"Set Data", "Get Data"}."Set Data", "Integer In"="Sample Rate") -> ()  [unwired: 9 in, 1 out]
        n131 = call <vilib>:"DAQmxBase Start Task.vi"("task/channels in"=w377, "error in"=w376) -> ("task out"=w375:refnum<k21>, "error out"=w374:errorcluster)  [unwired: 12 in]
      }
      frame "Exit" {
      }
    }
    n132 = Get Notifier Status(notifier=w319, error in (no error)=w318) -> (current notification=w320:bool)  [unwired: 4 out]
    n133 = Or(x=w330, y=w320) -> (x .or. y?=w321:bool)
  }
  n134 = Release Queue(queue=w26, error in (no error)=w25) -> ()  [unwired: 1 in, 3 out]
  n135 = Release Queue(queue=w24, error in (no error)=w23) -> (error out=w15:errorcluster)  [unwired: 1 in, 2 out]
  n136 = call <vilib>:"DAQmxBase Clear Task.vi"("task in"=w17, "error in"=w16) -> ("error out"=w14:errorcluster)  [unwired: 13 in]
  n137 = Merge Errors(w15, w14) -> (w13:errorcluster)
  n138 = call <vilib>:"Simple Error Handler.vi"("error in (no error)"=w13) -> ()  [unwired: 4 in, 5 out]
